vi "Get Application Extension.vi"(8 "error in (no error)":errorcluster caption="错误输入（无错误）", 11 "Gif Image 输入":refnum<class "Gif Image.lvclass"> caption="DNL_LabVIEW Object in") -> (0 "error out":errorcluster caption="错误输出", 2 "Application Extension":T1 {"Application Extension Labe(1)l" format="0x%02x" items=["Image Seperator"=44, "Extension Introducer"=33, "Graphic Control Label"=249, "Comment Label"=254, "PlainText Label"=1, "Gif Trailor"=59, "Application Label"=255]; "ID(1)" format="0x%02x" items=["Image Seperator"=44, "Extension Introducer"=33, "Graphic Control Label"=249, "Comment Label"=254, "PlainText Label"=1, "Gif Trailor"=59, "Application Label"=255]}, 3 "Gif Image 输出":refnum<class "Gif Image.lvclass"> caption="DNL_LabVIEW Object out")   [LabVIEW 2012, in "Picture Box Tools.lvlib" / "Gif Image.lvclass"]
uses:
  Gif Image.lvclass
  Control/Application Extension.ctl
  Control/ID Charactor.ctl
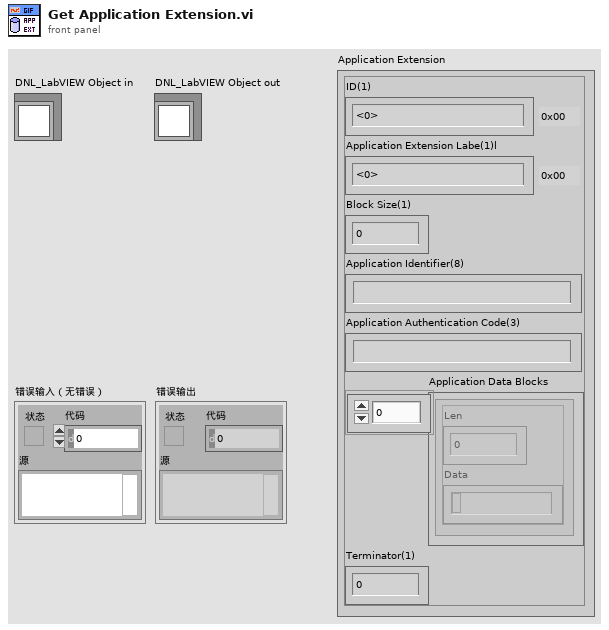
[diagram p1: front panel]
types:
  T1 = typedef "Picture Box Tools.lvlib/Gif Image.lvclass/Application Extension.ctl" = cluster{"ID(1)":T2, "Application Extension Labe(1)l":T2, "Block Size(1)":u8, "Application Identifier(8)":string, "Application Authentication Code(3)":string, "Application Data Blocks":cluster{"Len":u8, "Data":string}[], "Terminator(1)":u8}
  T2 = typedef "Picture Box Tools.lvlib/Gif Image.lvclass/ID Charactor.ctl" = u8
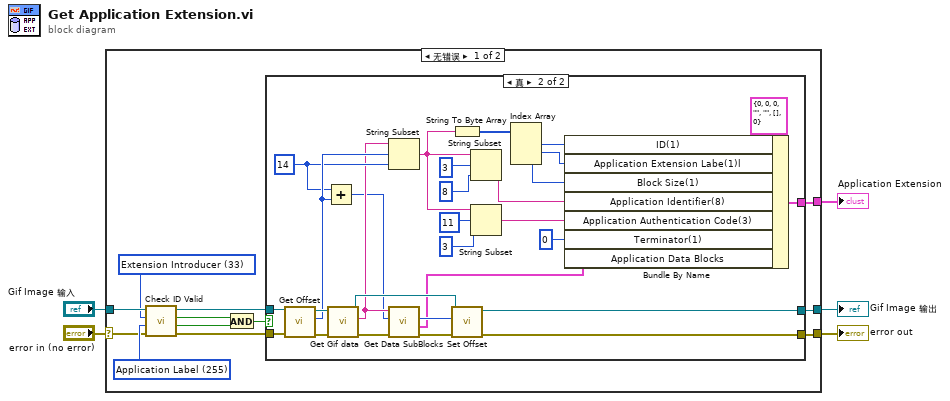
[diagram p0: block diagram]
diagram:
  n1 = case shown="无错误" "error in (no error)" {
    selector: "error in (no error)" -> [w9 w50]
    tunnel: [w7 w50] -> w4
    tunnel: [w10 _] -> w2
    tunnel: "Gif Image 输入" -> [w17 w49]
    tunnel: [w6 w49] -> w1
    frame No Error {
      w15 = T2 255 items=["Image Seperator"=44, "Extension Introducer"=33, "Graphic Control Label"=249, "Comment Label"=254, "PlainText Label"=1, "Gif Trailor"=59, "Application Label"=255] ("Label")
      w16 = T2 33 items=["Image Seperator"=44, "Extension Introducer"=33, "Graphic Control Label"=249, "Comment Label"=254, "PlainText Label"=1, "Gif Trailor"=59, "Application Label"=255] ("ID")
      n2 = call "Check ID Valid.vi"("error in (no error)"=w9, "Label"=w15, "ID"=w16, "Gif Image 输入"=w17) -> ("error out"=w8:errorcluster, "Label Valid"=w13:bool, "ID Valid"=w14:bool, "Gif Image 输出"=w11:refnum<class "Gif Image.lvclass">)  [unwired: 4 in]
      n3 = And(x=w14, y=w13) -> (x .and. y?=w12:bool)
      n4 = case shown="真" w12 {
        tunnel: w11 -> [w18 w48]
        tunnel: [_ w39] -> w10
        tunnel: w8 -> [w19 w47]
        tunnel: [w19 w35] -> w7
        tunnel: [w18 w34] -> w6
        frame False {
        }
        frame True {
          w37 = 14 ("长度（剩余）")
          n5 = call "Get Offset.vi"("error in (no error)"=w47, "Gif Image输入"=w48) -> ("error out"=w46:errorcluster, "Offset"=w38:i32, "Gif Image输出"=w45:refnum<class "Gif Image.lvclass">)  [unwired: 7 in]
          n6 = Add(x=w37, y=w38) -> (x+y=w22:i32)
          n7 = call "Get Gif data.vi"("error in (no error)"=w46, "Gif Image输入"=w45) -> ("error out"=w26:errorcluster, "Gif data"=w24:string, "Gif Image输出"=w36:refnum<class "Gif Image.lvclass">)  [unwired: 7 in]
          n8 = String Subset(string=w24, offset (0)=w38, length (rest)=w37) -> (substring=w31:string)
          n9 = call "Get Data SubBlocks.vi"("错误输入"=w26, "Offset In"=w22, "Gif data in"=w24) -> ("错误输出"=w25:errorcluster, "Data Blocks"=w20:cluster{"Len":u8, "Gif data Out":string}[], "Offset Out"=w23:i32)  [unwired: 5 in, 1 out]
          n10 = String To Byte Array(string=w31) -> (unsigned byte array=w40:u8[])
          n11 = call "Set Offset.vi"("error in (no error)"=w25, "Offset"=w23, "Gif Image输入"=w36) -> ("error out"=w35:errorcluster, "Gif Image输出"=w34:refnum<class "Gif Image.lvclass">)  [unwired: 7 in]
          n12 = String Subset(string=w31, offset (0)=3 ("索引"), length (rest)=8 ("长度")) -> (substring=w27:string)
          n13 = String Subset(string=w31, offset (0)=11 ("索引"), length (rest)=3 ("长度")) -> (substring=w28:string)
          n14 = Index Array(array=w40) -> (element #1=w43:u8, element #2=w42:u8, element #3=w41:u8)  [unwired: 3 in]
          n15 = Bundle By Name(cluster=T1 {"ID(1)"=0, "Application Extension Labe(1)l"=0, "Block Size(1)"=0, "Application Identifier(8)"="", "Application Authentication Code(3)"="", "Application Data Blocks"=[], "Terminator(1)"=0} ("Application Extension"), "ID(1)"=w43, "Application Extension Labe(1)l"=w42, "Block Size(1)"=w41, "Application Identifier(8)"=w27, "Application Authentication Code(3)"=w28, "Terminator(1)"=u8 0, "Application Data Blocks"=w20) -> (w39:T1)
        }
      }
    }
    frame Error {
    }
  }
  "error out" <- w4
  "Application Extension" <- w2
  "Gif Image 输出" <- w1
